vi "processCmd.vi"(8 "error in (no error)":errorcluster, 10 "tcpPacket":T1, 11 "tcpServer in":refnum<class "TcpServer.lvclass">) -> (0 "error out":errorcluster, 3 "tcpServer out":refnum<class "TcpServer.lvclass">)   [LabVIEW 2018, in "TcpServer.lvclass"]
doc: "Process the incomming command.\n\nNOTE: Do not call this directly.This is for internal use only."
uses:
  TcpServer.lvclass
  typedef/tcpPacketTypeDef.ctl
  TcpServer.lvclass/TcpServer.ctl
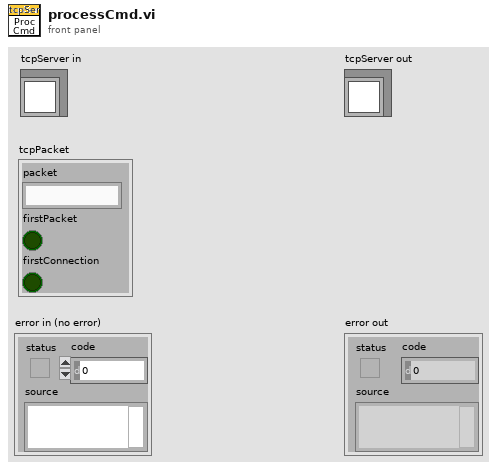
[diagram p1: front panel]
types:
  T1 = typedef "TcpServer.lvclass/tcpPacketTypeDef.ctl" = cluster{"packet":string, "firstPacket":bool, "firstConnection":bool}
  T2 = typedef "TcpServer.lvclass/userEventsTypeDef.ctl" = cluster{"TcpServer":refnum<user-event>, "Cmd":refnum<user-event>, "CmdStatus":refnum<user-event>, "Event":refnum<user-event>}
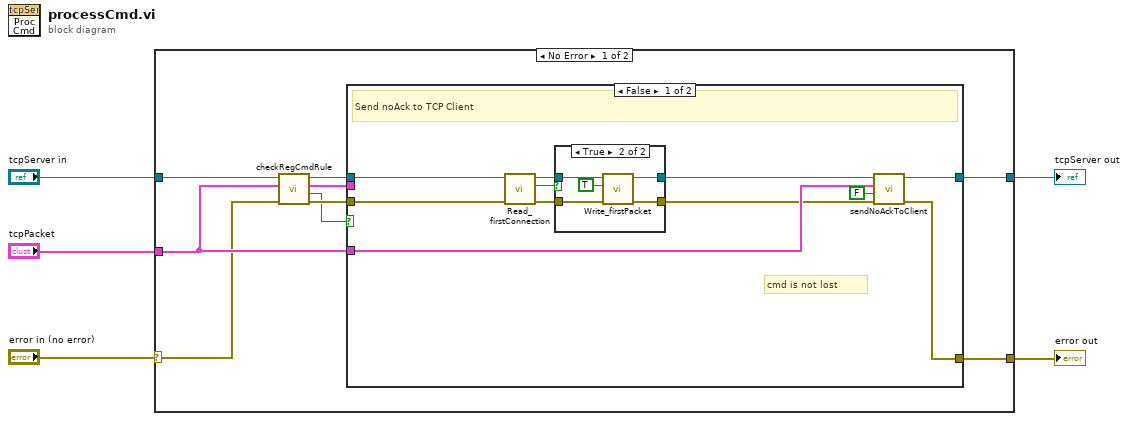
[diagram p0: block diagram]
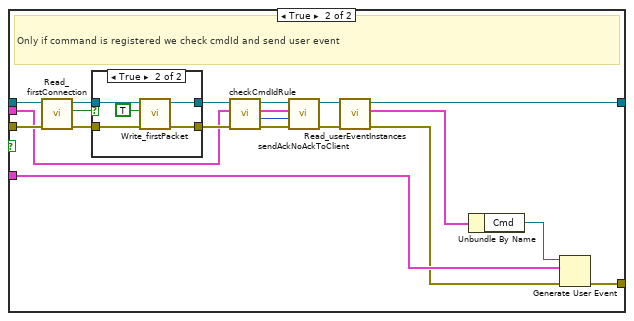
[diagram p3: hidden frame]
diagram:
  n1 = case shown="No Error" "error in (no error)" {
    selector: "error in (no error)" -> [w8 w61]
    tunnel: [w6 w61] -> w4
    tunnel: [w7 w60] -> w2
    tunnel: "tcpServer in" -> [w10 w60]
    tunnel: "tcpPacket" -> [w9 _]
    frame No Error {
      n2 = call "checkRegCmdRule.vi"("error in (no error)"=w8, "packetConnID"=w9, "tcpServer in"=w10) -> ("error out"=w12:errorcluster, "regCmd?"=w11:bool, "packetConnID"=w13:T1, "tcpServer out"=w14:refnum<class "TcpServer.lvclass">)  [unwired: 5 in]
      n3 = case shown="False" w11 {
        tunnel: [w24 w50] -> w7
        tunnel: [w25 w49] -> w6
        tunnel: w9 -> [w23 w48]
        tunnel: w14 -> [w22 w38]
        tunnel: w13 -> [_ w33]
        tunnel: w12 -> [w18 w40]
        frame False {
          # "cmd is not lost"
          # "Send noAck to TCP Client"
          n4 = call "Read_firstConnection.vi"("error in (no error)"=w18, "TcpServer in"=w22) -> ("error out"=w19:errorcluster, "firstConnection"=w20:bool, "TcpServer out"=w21:refnum<class "TcpServer.lvclass">)  [unwired: 7 in]
          n5 = case shown="True" w20 {
            tunnel: w19 -> [w26 w32]
            tunnel: [w26 w31] -> w16
            tunnel: w21 -> [w27 w30]
            tunnel: [w27 w29] -> w17
            frame False {
            }
            frame True {
              n6 = call "Write_firstPacket.vi"("error in (no error)"=w32, "firstPacket"=TRUE, "TcpServer in"=w30) -> ("error out"=w31:errorcluster, "TcpServer out"=w29:refnum<class "TcpServer.lvclass">)  [unwired: 7 in]
            }
          }
          n7 = call "sendNoAckToClient.vi"("error in (no error)"=w16, "cmdLost"=FALSE, "tcpPacket"=w23, "tcpServer in"=w17) -> ("error out"=w25:errorcluster, "tcpServer out"=w24:refnum<class "TcpServer.lvclass">)  [unwired: 6 in]
        }
        frame True {
          # "Only if command is registered we check cmdId and send user event"
          n8 = call "Read_firstConnection.vi"("error in (no error)"=w40, "TcpServer in"=w38) -> ("error out"=w39:errorcluster, "firstConnection"=w34:bool, "TcpServer out"=w36:refnum<class "TcpServer.lvclass">)  [unwired: 7 in]
          n9 = case shown="True" w34 {
            tunnel: w39 -> [w53 w59]
            tunnel: [w53 w58] -> w37
            tunnel: w36 -> [w54 w57]
            tunnel: [w54 w56] -> w35
            frame False {
            }
            frame True {
              n10 = call "Write_firstPacket.vi"("error in (no error)"=w59, "firstPacket"=TRUE, "TcpServer in"=w57) -> ("error out"=w58:errorcluster, "TcpServer out"=w56:refnum<class "TcpServer.lvclass">)  [unwired: 7 in]
            }
          }
          n11 = call "checkCmdIdRule.vi"("error in (no error)"=w37, "packetConnID"=w33, "tcpServer in"=w35) -> ("error out"=w46:errorcluster, "ackIterations"=w45:i32, "packetConnID"=w44:T1, "tcpServer out"=w47:refnum<class "TcpServer.lvclass">)  [unwired: 5 in]
          n12 = call "sendAckNoAckToClient.vi"("error in (no error)"=w46, "ackIterations"=w45, "tcpPacket"=w44, "tcpServer in"=w47) -> ("error out"=w51:errorcluster, "tcpServer out"=w52:refnum<class "TcpServer.lvclass">)  [unwired: 6 in]
          n13 = call "Read_userEventInstances.vi"("error in (no error)"=w51, "tcpServer in"=w52) -> ("error out"=w41:errorcluster, "UserEvents"=w42:T2, "tcpServer out"=w50:refnum<class "TcpServer.lvclass">)  [unwired: 7 in]
          n14 = Unbundle By Name(w42) -> ("Cmd"=w43:refnum<user-event>)
          n15 = Generate User Event(user event=w43, event data cluster=w48, error in=w41) -> (error out=w49:errorcluster)  [unwired: 1 in, 1 out]
        }
      }
    }
    frame Error {
    }
  }
  "error out" <- w4
  "tcpServer out" <- w2
